vi "Read Modulation.vi"(8 "error in (no error)":errorcluster, 11 "Change Laser Modulation in":refnum<class "Change Laser Modulation.lvclass">) -> (0 "error out":errorcluster, 2 "Modulation":T1, 3 "Change Laser Modulation out":refnum<class "Change Laser Modulation.lvclass">)   [LabVIEW 2014, in "Change Laser Modulation.lvclass"]
uses:
  Change Laser Modulation.lvclass
  reusable/PAS/Controls/Modulation Type.ctl
  Change Laser Modulation.lvclass/Change Laser Modulation.ctl
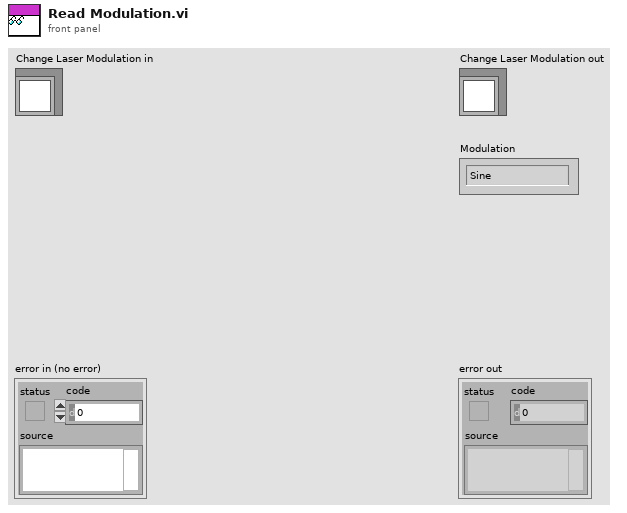
[diagram p1: front panel]
types:
  T1 = typedef "Modulation Type.ctl" = enum16{"Sine", "Square"}
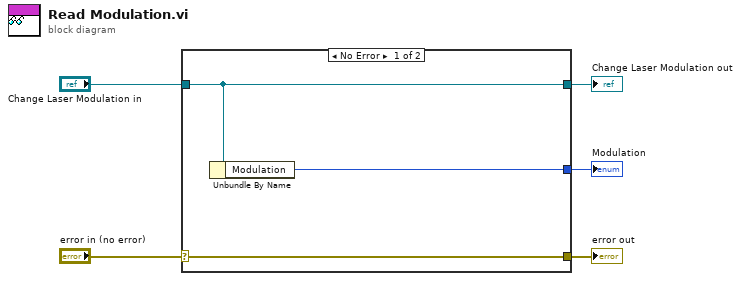
[diagram p0: block diagram]
diagram:
  n1 = case shown="No Error" "error in (no error)" {
    selector: "error in (no error)" -> [w8 w9]
    tunnel: [w8 w9] -> w4
    tunnel: [w7 w10] -> w2
    tunnel: "Change Laser Modulation in" -> [w7 w10]
    tunnel: [w6 _] -> w1
    frame No Error {
      n2 = Unbundle By Name(w7) -> ("Modulation"=w6:T1)
    }
    frame Error {
    }
  }
  "error out" <- w4
  "Change Laser Modulation out" <- w2
  "Modulation" <- w1
